vi "ProdaNG.Oracle.GetInstances.vi"(8 "error in (no error)":errorcluster, 10 "Tnsnames path":path) -> (0 "error out":errorcluster, 1 "Instances Names":string[](array[string]), 2 "Instances":T1[](array[typedef]))   [LabVIEW 2016]
uses:
  ProdaNG.Oracle.InstanceData.ctl
panel:
  out "dbg":string[](array[string])
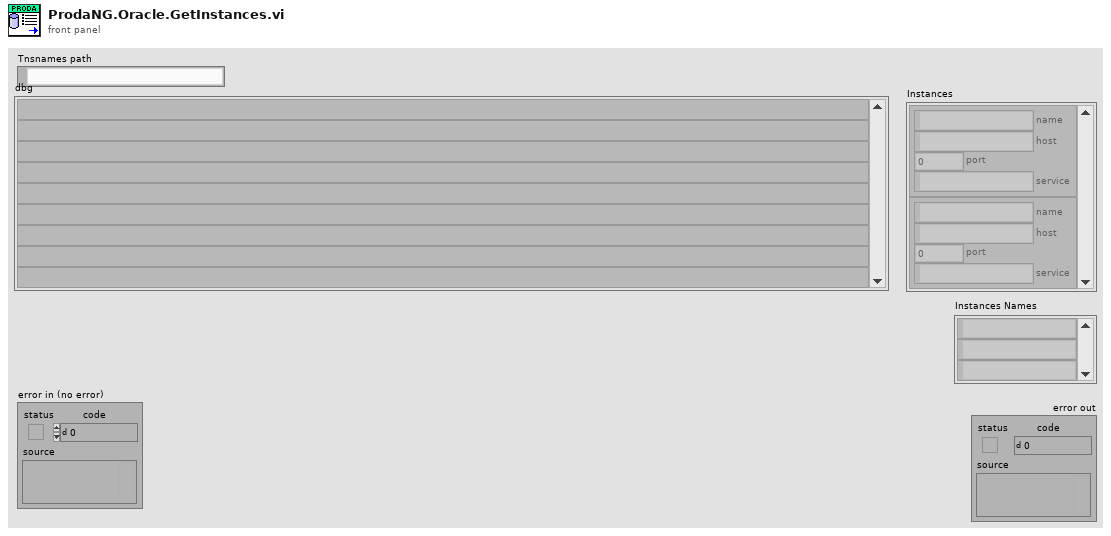
[diagram p1: front panel]
types:
  T1 = typedef "ProdaNG.Oracle.InstanceData.ctl" = cluster{"name":string, "host":string, "port":u16, "service":string}
  T2 = enum16{"read/write", "read-only", "write-only", "write-only (truncate)"}
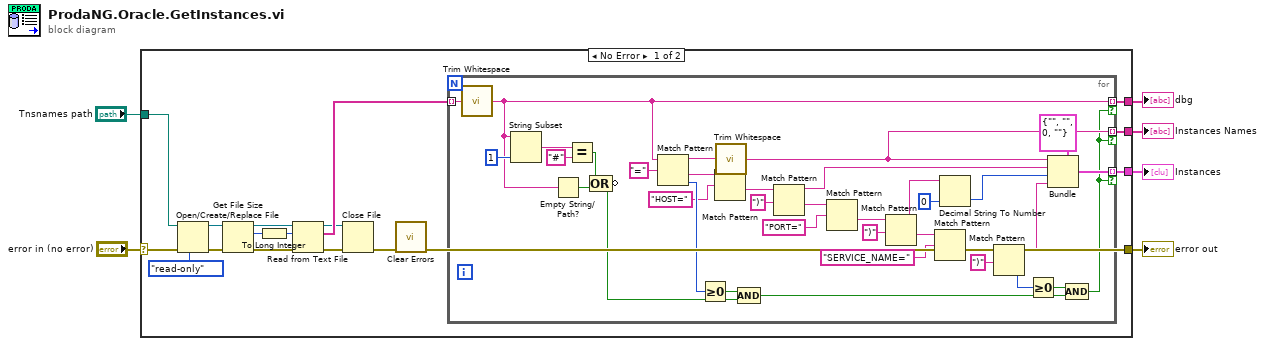
[diagram p0: block diagram]
diagram:
  n1 = case shown="No Error" "error in (no error)" {
    selector: "error in (no error)" -> [w15 w60]
    tunnel: [w8 w60] -> w6
    tunnel: "Tnsnames path" -> [w16 _]
    tunnel: [w10 _] -> w3
    tunnel: [w9 _] -> w2
    tunnel: [w7 _] -> w1
    frame No Error {
      n2 = Open/Create/Replace File(file path (use dialog)=w16, error in=w15, access (0:read/write)=T2."read-only" ("open mode (0)")) -> (refnum out=w21:refnum<file>, error out=w20:errorcluster)  [unwired: 4 out]
      n3 = Get File Size(file=w21, error in=w20) -> (refnum out=w22:refnum<file>, size (in bytes)=w18:i64, 0:w23:errorcluster)
      n4 = To Long Integer(number=w18) -> (32bit integer=w17:i32)
      n5 = Read from Text File(file (use dialog)=w22, count=w17, error in=w23) -> (refnum out=w13:refnum<file>, text=w14:string[], error out=w12:errorcluster)  [unwired: 1 in, 1 out]
      n6 = Close File(refnum=w13, error in=w12) -> (error out=w11:errorcluster)  [unwired: 1 out]
      n7 = call <vilib>:"Clear Errors.vi"("error in (no error)"=w11) -> ("error out"=w8:errorcluster)  [unwired: 5 in, 1 out]
      n8 = for {
        tunnel: w14 -> [w59] mode=indexing
        tunnel: [w30] -> w9 mode=indexing if=w24
        tunnel: [w32] -> w10 mode=indexing if=w24
        tunnel: [w25] -> w7 mode=indexing if=w24
        n9 = call <vilib>:"Trim Whitespace.vi"("string"=w59) -> ("trimmed string"=w30:string)  [unwired: 1 in]
        n10 = String Subset(string=w30, length (rest)=1 ("length (rest)")) -> (substring=w55:string)  [unwired: 1 in]
        n11 = Empty String/Path?(string/path=w30) -> (empty?=w58:bool)
        n12 = Equal?(x=w55, y="#") -> (x = y?=w54:bool)
        n13 = Compound Arithmetic op=OR(w54, w58) -> (invert w50:bool)
        n14 = Match Pattern(string=w30, regular expression="=") -> (before substring=w52:string, after substring=w48:string, offset past match=w33:i32)  [unwired: 1 in, 1 out]
        n15 = Greater Or Equal To 0?(x=w33) -> (x >= 0?=w51:bool)
        n16 = Match Pattern(string=w48, regular expression="HOST=") -> (after substring=w47:string)  [unwired: 1 in, 3 out]
        n17 = call <vilib>:"Trim Whitespace.vi"("string"=w52) -> ("trimmed string"=w25:string)  [unwired: 1 in]
        n18 = Compound Arithmetic op=AND(w51, w50) -> (w26:bool)
        n19 = Match Pattern(string=w47, regular expression=")") -> (before substring=w45:string, after substring=w42:string)  [unwired: 1 in, 2 out]
        n20 = Match Pattern(string=w42, regular expression="PORT=") -> (after substring=w43:string)  [unwired: 1 in, 3 out]
        n21 = Match Pattern(string=w43, regular expression=")") -> (before substring=w41:string, after substring=w35:string)  [unwired: 1 in, 2 out]
        n22 = Match Pattern(string=w35, regular expression="SERVICE_NAME=") -> (after substring=w37:string)  [unwired: 1 in, 3 out]
        n23 = Decimal String To Number(string=w41, default (0L)=u16 0 ("default (0 I32)")) -> (number=w39:u16)  [unwired: 1 in, 1 out]
        n24 = Match Pattern(string=w37, regular expression=")") -> (before substring=w29:string, offset past match=w27:i32)  [unwired: 1 in, 2 out]
        n25 = Greater Or Equal To 0?(x=w27) -> (x >= 0?=w28:bool)
        n26 = Bundle(cluster=T1 {"name"="", "host"="", "port"=0, "service"=""} ("InstanceData"), "name"=w25, "host"=w45, "port"=w39, "service"=w29) -> (w32:T1)
        n27 = Compound Arithmetic op=AND(w28, w26) -> (w24:bool)
      }
    }
    frame Error {
    }
  }
  "error out" <- w6
  "Instances" <- w3
  "dbg" <- w2
  "Instances Names" <- w1
